vi "RemainingTime.vi"(1 "Timings":dbl[][](array[numeric])=[[2417234066.0, 52858.0]] format="%^_3e", 2 "sweep_dim":u64[](array[numeric]), 3 "Count":u64) -> (0 "Remaning time (min)":dbl)   [LabVIEW 2013]
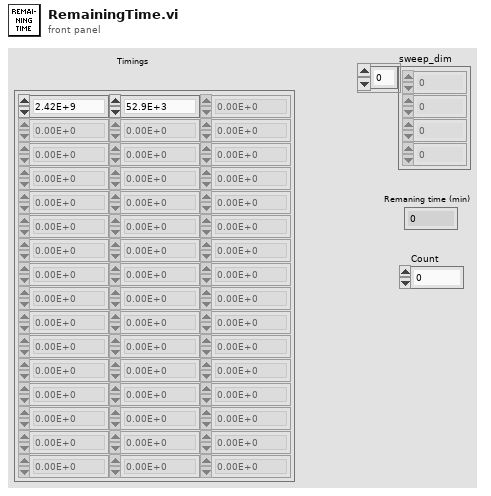
[diagram p1: front panel]
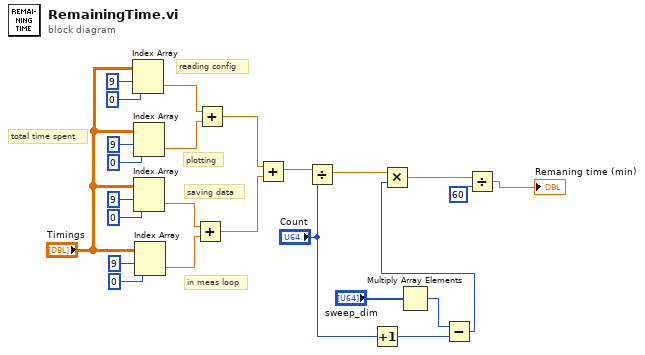
[diagram p0: block diagram]
diagram:
  # "in meas loop"
  # "saving data"
  # "plotting"
  # "reading config"
  # "total time spent"
  n1 = Index Array(array="Timings", index (row)=9, index (col)=0) -> (element=w16:dbl)
  n2 = Index Array(array="Timings", index (row)=9, index (col)=0) -> (element=w15:dbl)
  n3 = Index Array(array="Timings", index (row)=9, index (col)=0) -> (element=w14:dbl)
  n4 = Index Array(array="Timings", index (row)=9, index (col)=0) -> (element=w13:dbl)
  n5 = Add(x=w14, y=w13) -> (x+y=w11:dbl)
  n6 = Add(x=w16, y=w15) -> (x+y=w12:dbl)
  n7 = Add(x=w12, y=w11) -> (x+y=w9:dbl)
  n8 = Divide(x=w9, y="Count") -> (x/y=w5:dbl)
  n9 = Increment(x="Count") -> (x+1=w2:u64)
  n10 = Multiply Array Elements(1:"sweep_dim") -> (0:w6:u64)
  n11 = Subtract(x=w6, y=w2) -> (x-y=w4:u64)
  n12 = Multiply(x=w5, y=w4) -> (x*y=w3:dbl)
  n13 = Divide(x=w3, y=60) -> (x/y=→"Remaning time (min)":dbl)
